vi "TSPopup.Lookup.vi"(8 "error in (no error)":errorcluster, 9 "Point":cluster{"X":i32, "Y":i32}, 10 "Ctl Refnum":refnum<vi>, 11 "TSPopup in":refnum<class "TSPopup.lvclass">) -> (0 "error out":errorcluster, 1 "In Bounds?":bool, 2 "Found":bool, 3 "TSPopup out":refnum<class "TSPopup.lvclass">, 4 "Cell Info (Call data)":T1, 5 "Popup Parameters":T3)   [LabVIEW 2016, in "TSPopup.lvlib" / "TSPopup.lvclass"]
doc: "Searches the registered controls for Popup Parameters (type) associated with the location that was clicked on. Search order is : Exact Cell, Entire Column, Entire Row, Entire Control.\n\n<B>Ctl Refnum</B> - Refnum of the control that was clicked on. This same reference should have been used to register parameters using \"TSPopup.Register.vi\"\n<B>Point</B> - Mouse coordinates of <B>Mouse Down?</B> Event.\n\n<B>Popup Parameters</B> - Parameters for showing the Type Sensitive Popup.\n<B>Found</B> - Indicates whether the clicked location had parameters registered.\n<B>In Bounds?</B> - Indicates whether the mouse click was within main area of control (not the label, caption, scrollbars, etc.).\n<B>Cell Info (Call data)</B> - This provides helpful information for editing the Popup Parameters and for sending as the Call Data.\n\nType Sensitive Popup \nCopyright © 2007, J. David Saunders\nAll rights reserved."
uses:
  <userlib>/TSPopup/TSPopup.lvclass
  <userlib>/TSPopup/TSPopup.Popup Call Parameters.ctl
  <userlib>/TSPopup/TSPopup.Data Type.ctl
  <userlib>/TSPopup/TSPopup.Grid.Cell Info.ctl
  <userlib>/TSPopup/TSPopup.lvclass/TSPopup.ctl
panel:
  # "Type Sensitive Popup \nCopyright © 2007, J. David Saunders\nAll rights reserved."
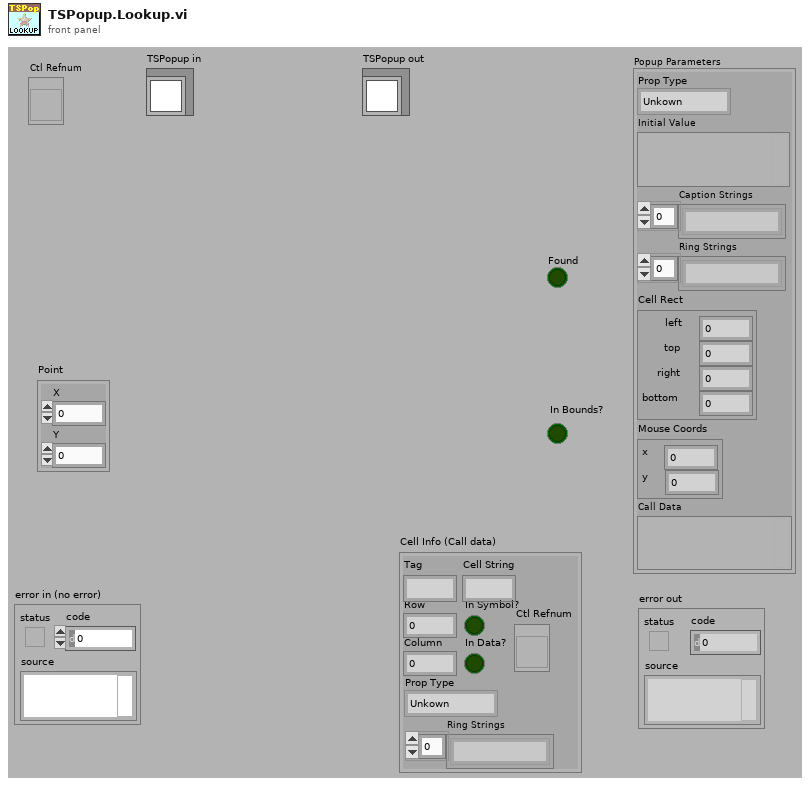
[diagram p1: front panel]
types:
  T1 = typedef "TSPopup.lvlib/TSPopup.lvclass/TSPopup.Grid.Cell Info.ctl" = cluster{"Tag":string, "Row":i32, "Column":i32, "In Symbol?":bool, "In Data?":bool, "Cell String":string, "Ctl Refnum":refnum<vi>, "Prop Type":T2, "Ring Strings":string[]}
  T2 = typedef "TSPopup.lvlib/TSPopup.lvclass/TSPopup.Data Type.ctl" = enum16{"Unkown", "NO POPUP", "String", "Integer", "Float", "Color", "Boolean", "Ring", "Captioned String", "Captioned Integer", "Button Color", "2 Int Cluster", "4 Int Cluster", "check"}
  T3 = typedef "TSPopup.lvlib/TSPopup.lvclass/TSPopup.Popup Call Parameters.ctl" = cluster{"Prop Type":T2, "Initial Value":variant, "Caption Strings":string[], "Ring Strings":string[], "Cell Rect":cluster{"left":i16, "top":i16, "right":i16, "bottom":i16}, "Mouse Coords":cluster{"x":i16, "y":i16}, "Call Data":variant}
  T4 = cluster{"left":i16, "top":i16, "right":i16, "bottom":i16}
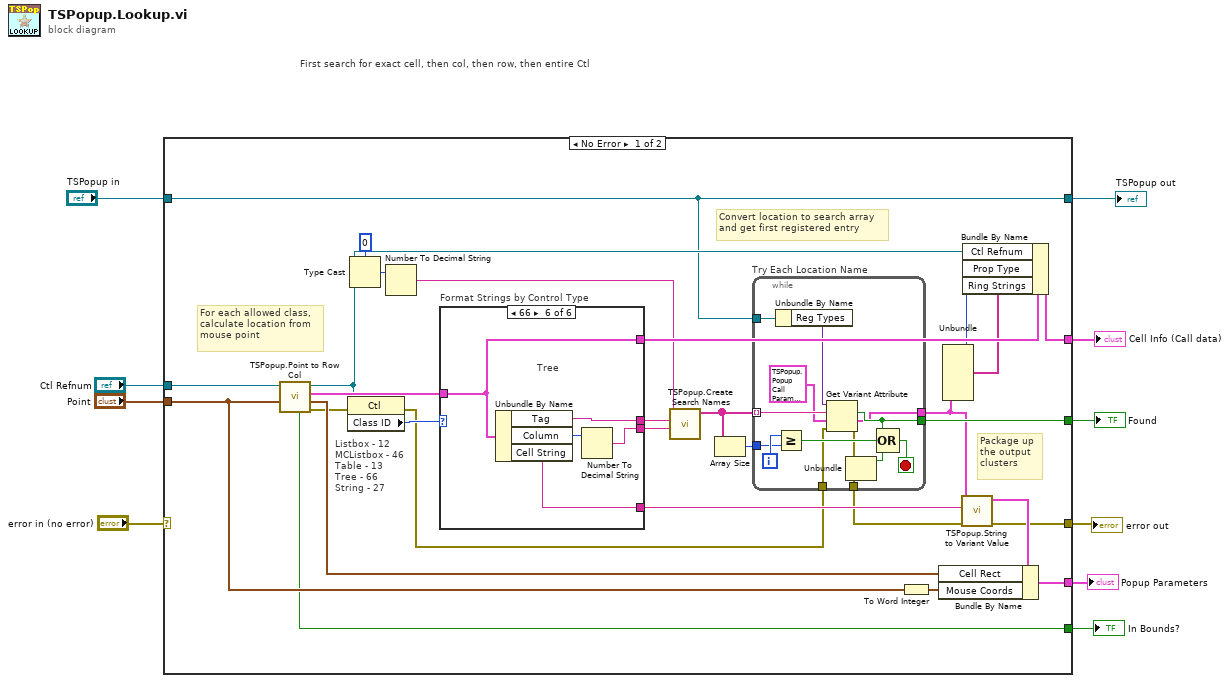
[diagram p0: block diagram]
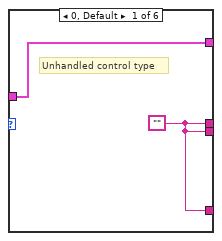
[diagram p2: hidden frame]
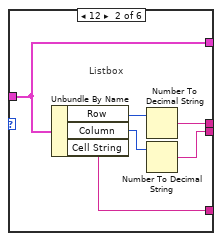
[diagram p3: hidden frame]
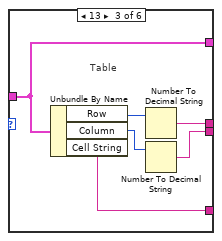
[diagram p4: hidden frame]
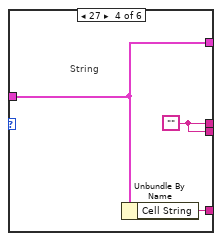
[diagram p5: hidden frame]
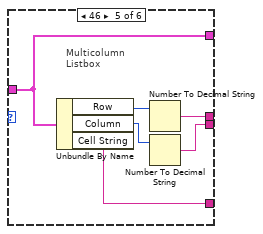
[diagram p6: hidden frame]
diagram:
  # "First search for exact cell, then col, then row, then entire Ctl"
  n1 = case shown="No Error" "error in (no error)" {
    selector: "error in (no error)" -> [_ w82]
    tunnel: [w21 w82] -> w8
    tunnel: "Ctl Refnum" -> [w20 _]
    tunnel: "Point" -> [w18 _]
    tunnel: [w34 _] -> w9
    tunnel: [w29 _] -> w7
    tunnel: [w15 _] -> w6
    tunnel: [w27 _] -> w10
    tunnel: "TSPopup in" -> [w11 w81]
    tunnel: [w11 w81] -> w1
    frame No Error {
      # "Package up\nthe output\nclusters"
      # "Convert location to search array\nand get first registered entry"
      # "For each allowed class,\ncalculate location from\nmouse point"
      # "Listbox - 12\nMCListbox - 46\nTable - 13\nTree - 66\nString - 27"
      n2 = call <userlib>:"TSPopup.Point to Row Col.vi"("Point"=w18, "Grid Ctl Reference In"=w20) -> ("error out"=w14:errorcluster, "Cell Rect Out"=w17:T4, "Cell Info Out"=w19:T1, "Grid Ctl Reference Out"=w12:refnum<vi>, "In Bounds?"=w15:bool)  [unwired: 5 in]
      n3 = property class="Ctl"(reference=w12, error in=w14) -> (error out=w13:errorcluster, "Class ID"=w39:u32)  [unwired: 1 out]
      n4 = Type Cast(type=0, x=w12) -> (*(type *) &x=w37:i32)
      n5 = Number To Decimal String(number=w37) -> (decimal integer string=w16:string)  [unwired: 1 in]
      n6 = case "Format Strings by Control Type" shown="66" w39 {
        tunnel: [w54 w59 w65 w69 w74 w80] -> w33
        tunnel: [w54 w57 w64 w69 w73 w78] -> w32
        tunnel: [w54 w56 w66 w68 w75 w77] -> w28
        tunnel: [w53 w55 w61 w67 w70 w76] -> w26
        tunnel: w19 -> [w53 w55 w61 w67 w70 w76]
        frame 0, Default {
          w54 = ""
          # "Unhandled control type"
        }
        frame 12 {
          # "Listbox"
          n7 = Unbundle By Name(w55) -> ("Row"=w60:i32, "Column"=w58:i32, "Cell String"=w56:string)
          n8 = Number To Decimal String(number=w60) -> (decimal integer string=w59:string)  [unwired: 1 in]
          n9 = Number To Decimal String(number=w58) -> (decimal integer string=w57:string)  [unwired: 1 in]
        }
        frame 13 {
          # "Table"
          n10 = Unbundle By Name(w61) -> ("Row"=w63:i32, "Column"=w62:i32, "Cell String"=w66:string)
          n11 = Number To Decimal String(number=w63) -> (decimal integer string=w65:string)  [unwired: 1 in]
          n12 = Number To Decimal String(number=w62) -> (decimal integer string=w64:string)  [unwired: 1 in]
        }
        frame 27 {
          w69 = ""
          # "String"
          n13 = Unbundle By Name(w67) -> ("Cell String"=w68:string)
        }
        frame 46 {
          # "Multicolumn\nListbox"
          n14 = Unbundle By Name(w70) -> ("Row"=w72:i32, "Column"=w71:i32, "Cell String"=w75:string)
          n15 = Number To Decimal String(number=w72) -> (decimal integer string=w74:string)  [unwired: 1 in]
          n16 = Number To Decimal String(number=w71) -> (decimal integer string=w73:string)  [unwired: 1 in]
        }
        frame 66 {
          # "Tree"
          n17 = Unbundle By Name(w76) -> ("Tag"=w80:string, "Column"=w79:i32, "Cell String"=w77:string)
          n18 = Number To Decimal String(number=w79) -> (decimal integer string=w78:string)  [unwired: 1 in]
        }
      }
      n19 = call <userlib>:"TSPopup.Create Search Names.vi"("Column String"=w32, "Tag or Row String"=w33, "Control Ref String"=w16) -> ("Search Names"=w36:string[])  [unwired: 8 in]
      n20 = Array Size(array=w36) -> (size(s)=w35:i32)
      n21 = while "Try Each Location Name" {
        tunnel: [w41] -> w25
        tunnel: w36 -> [w46] mode=indexing
        tunnel: w35 -> [w51]
        tunnel: [w43] -> w34
        tunnel: w13 -> [w45]
        tunnel: [w44] -> w22
        tunnel: w11 -> [w47]
        i -> [w52]
        stop <- w48 stop-if-true
        n22 = Unbundle By Name(w47) -> ("Reg Types"=w40:variant)
        n23 = Greater Or Equal?(x=w52, y=w51) -> (x >= y?=w50:bool)
        n24 = Get Variant Attribute(Variant=w40, name=w46, default value (empty Variant)=T3 {"Prop Type"=enum."Unkown", "Initial Value"=variant, "Caption Strings"=[], "Ring Strings"=[], "Cell Rect"={"left"=0, "top"=0, "right"=0, "bottom"=0}, "Mouse Coords"={"x"=0, "y"=0}, "Call Data"=variant} ("Popup Parameters 2"), error in=w45) -> (found=w43:bool, value=w41:T3, error out=w44:errorcluster)  [unwired: 1 out]
        n25 = Unbundle(w44) -> ("status"=w49:bool)  [unwired: 2 out]
        n26 = Compound Arithmetic op=OR(w43, w50, w49) -> (w48:bool)
      }
      n27 = To Word Integer(number=w18) -> (16bit integer=w31:cluster{"X":i16, "Y":i16})
      n28 = Unbundle(w25) -> ("Prop Type"=w23:T2, "Ring Strings"=w24:string[])  [unwired: 5 out]
      n29 = call <userlib>:"TSPopup.String to Variant Value.vi"("error in (no error)"=w22, "Cell String"=w28, "Popup Parameters"=w25) -> ("error out"=w21:errorcluster, "Popup Parameters out"=w30:T3)  [unwired: 6 in, 1 out]
      n30 = Bundle By Name(cluster=w30, "Cell Rect"=w17, "Mouse Coords"=w31) -> (w29:T3)
      n31 = Bundle By Name(cluster=w26, "Ctl Refnum"=w12, "Prop Type"=w23, "Ring Strings"=w24) -> (w27:T1)
    }
    frame Error {
    }
  }
  "error out" <- w8
  "Found" <- w9
  "In Bounds?" <- w6
  "Popup Parameters" <- w7
  "Cell Info (Call data)" <- w10
  "TSPopup out" <- w1
